vi "lijnvolgen.vi"() -> ()   [LabVIEW 2019]
panel:
  in  "stop":bool
  out "wat doet hij":string
  in  "bepaalde input op tijdstip t":dbl[](array[numeric])
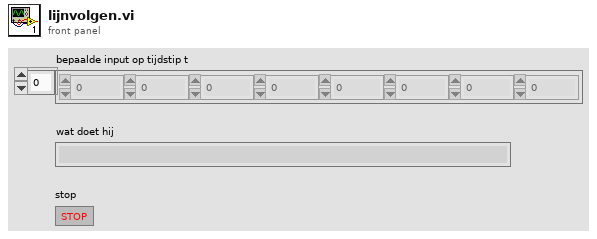
[diagram p1: front panel]
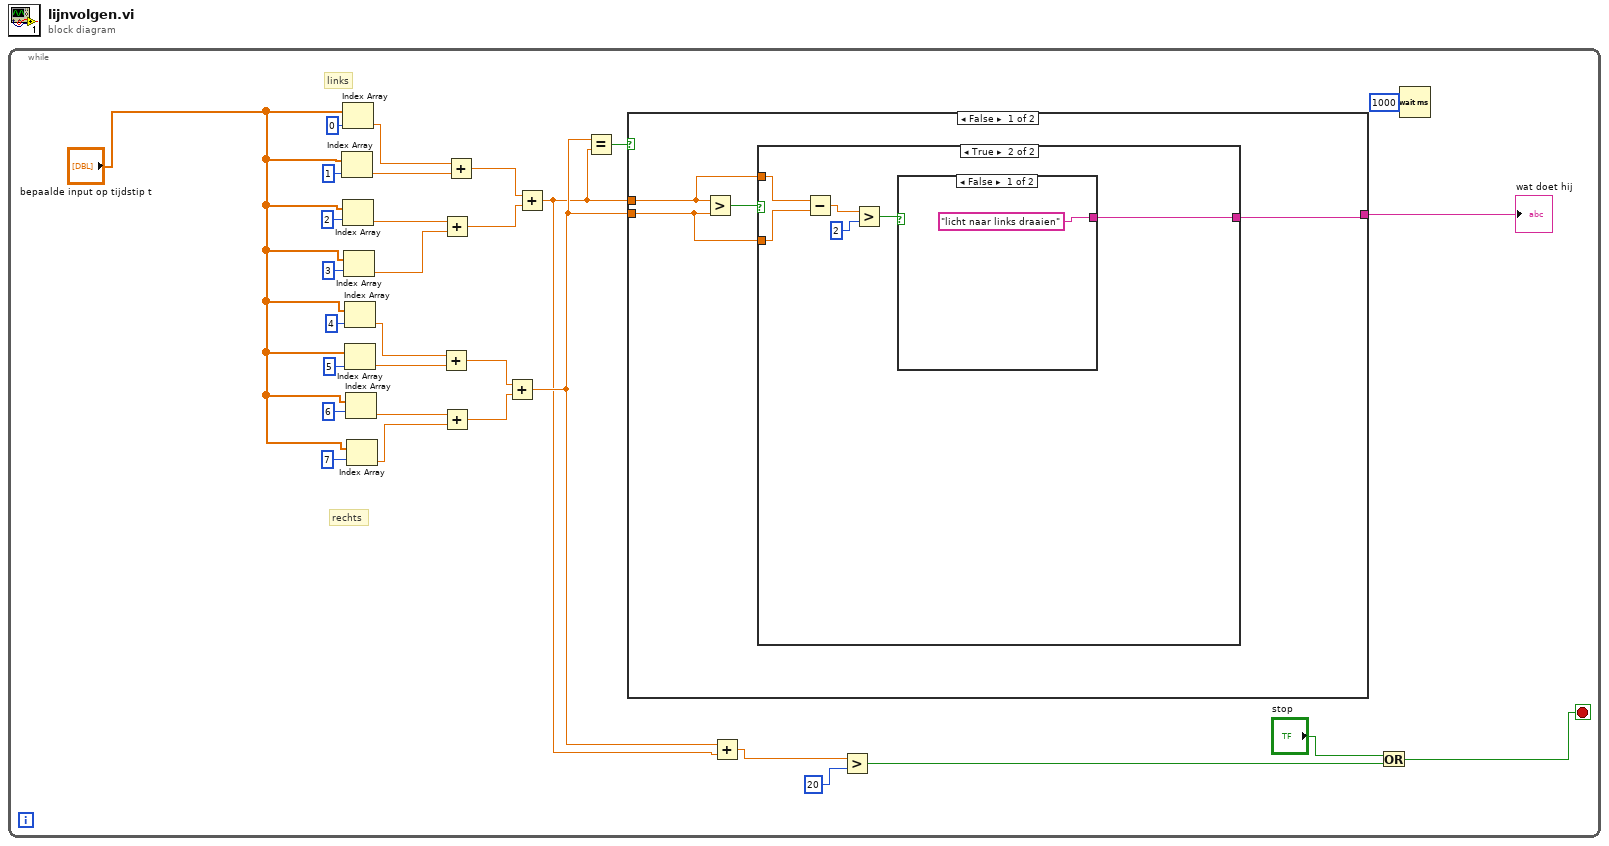
[diagram p0: block diagram]
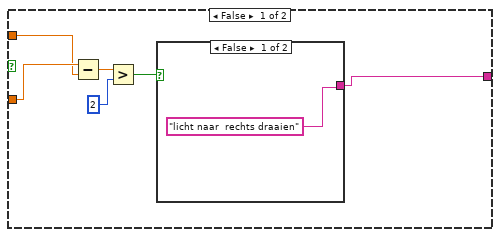
[diagram p2: hidden frame]
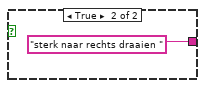
[diagram p3: hidden frame]
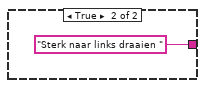
[diagram p4: hidden frame]
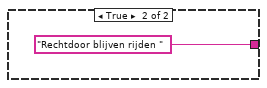
[diagram p5: hidden frame]
diagram:
  n1 = while {
    stop <- w1 stop-if-true
    # "rechts"
    # "links"
    n2 = Index Array(array="bepaalde input op tijdstip t", index=1) -> (element=w15:dbl)
    n3 = Index Array(array="bepaalde input op tijdstip t", index=0) -> (element=w16:dbl)
    n4 = Index Array(array="bepaalde input op tijdstip t", index=2) -> (element=w13:dbl)
    n5 = Index Array(array="bepaalde input op tijdstip t", index=3) -> (element=w14:dbl)
    n6 = Index Array(array="bepaalde input op tijdstip t", index=4) -> (element=w20:dbl)
    n7 = Index Array(array="bepaalde input op tijdstip t", index=5) -> (element=w19:dbl)
    n8 = Index Array(array="bepaalde input op tijdstip t", index=6) -> (element=w21:dbl)
    n9 = Index Array(array="bepaalde input op tijdstip t", index=7) -> (element=w22:dbl)
    n10 = Add(x=w20, y=w19) -> (x+y=w18:dbl)
    n11 = Add(x=w13, y=w14) -> (x+y=w11:dbl)
    n12 = Add(x=w21, y=w22) -> (x+y=w17:dbl)
    n13 = Add(x=w16, y=w15) -> (x+y=w12:dbl)
    n14 = Add(x=w18, y=w17) -> (x+y=w7:dbl)
    n15 = Add(x=w12, y=w11) -> (x+y=w6:dbl)
    n16 = Equal?(x=w7, y=w6) -> (x = y?=w10:bool)
    n17 = case shown="False" w10 {
      tunnel: w6 -> [w34 _]
      tunnel: [w32 "Rechtdoor blijven rijden "] -> w9
      tunnel: w7 -> [w33 _]
      frame False {
        n18 = Greater?(x=w34, y=w33) -> (0:w35:bool)
        n19 = case shown="True" w35 {
          tunnel: w34 -> [w40 w49]
          tunnel: w33 -> [w41 w48]
          tunnel: [w36 w44] -> w32
          frame False {
            n20 = Subtract(x=w41, y=w40) -> (x-y=w39:dbl)
            n21 = Greater?(x=w39, y=2) -> (0:w37:bool)
            n22 = case shown="False" w37 {
              tunnel: ["licht naar  rechts draaien" "sterk naar rechts draaien "] -> w36
              frame False {
              }
              frame True {
              }
            }
          }
          frame True {
            n23 = Subtract(x=w49, y=w48) -> (x-y=w47:dbl)
            n24 = Greater?(x=w47, y=2) -> (0:w45:bool)
            n25 = case shown="False" w45 {
              tunnel: ["licht naar links draaien" "Sterk naar links draaien "] -> w44
              frame False {
              }
              frame True {
              }
            }
          }
        }
      }
      frame True {
      }
    }
    "wat doet hij" <- w9
    n26 = Add(x=w7, y=w6) -> (x+y=w4:dbl)
    n27 = Greater?(x=w4, y=20) -> (0:w3:bool)
    n28 = Or(x="stop", y=w3) -> (x .or. y?=w1:bool)
    n29 = Wait (ms)(milliseconds to wait=1000) -> ()  [unwired: 1 out]
  }
